vi "Joystick Curve Linear.vi"(9 "Joystick Input":dbl, 10 "Encoder Input":dbl) -> (2 "Motor Output":dbl)   [LabVIEW 2011]
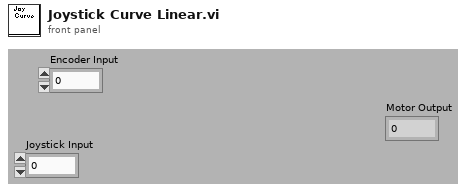
[diagram p1: front panel]
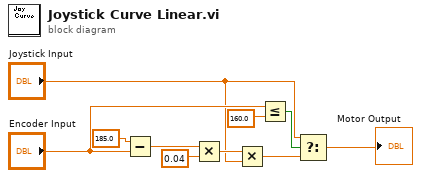
[diagram p0: block diagram]
diagram:
  n1 = Subtract(x=185.0, y="Encoder Input") -> (x-y=w9:dbl)
  n2 = Multiply(x=w9, y=0.04) -> (x*y=w7:dbl)
  n3 = Multiply(x=w7, y="Joystick Input") -> (x*y=w2:dbl)
  n4 = Less Or Equal?(x="Encoder Input", y=160.0) -> (x <= y?=w4:bool)
  n5 = Select(t="Joystick Input", s=w4, f=w2) -> (s? t:f=→"Motor Output":dbl)
